vi "Get CustomDevice Reference.vi"(8 "error in":errorcluster, 11 "Node Ptr":T1 format="%.0x") -> (0 "error out":errorcluster, 2 "Custom Device":refnum<k24>, 3 "Node Ptr":T1 format="%.0x")   [LabVIEW 2026, in "Template System Explorer.lvlib"]
uses:
  Template System Explorer.lvlib
  <vilib>/NI VeriStand/Custom Device API/Custom Device Item Ref.ctl
  NationalInstruments.VeriStand.SystemDefinitionAPI
  <vilib>/NI VeriStand/Custom Device API/Custom Device API.lvlib
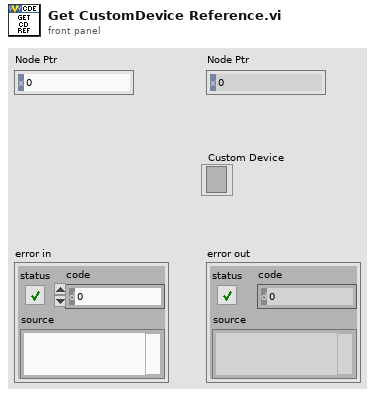
[diagram p1: front panel]
types:
  T1 = typedef "Custom Device API.lvlib/Custom Device Item Ref.ctl" = u64
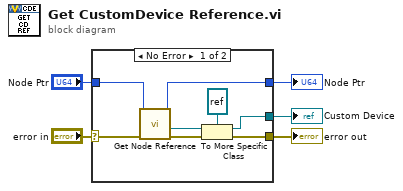
[diagram p0: block diagram]
diagram:
  n1 = case shown="No Error" "error in" {
    selector: "error in" -> [w10 w15]
    tunnel: [w9 w15] -> w4
    tunnel: "Node Ptr" -> [w7 w14]
    tunnel: [w8 w14] -> w2
    tunnel: [w11 _] -> w1
    frame No Error {
      n2 = call "Get Node Reference.vi"("error in"=w10, "Node Ptr"=w7) -> ("error out"=w13:errorcluster, "Base Node"=w6:refnum<k24>, "Node Ptr"=w8:T1)  [unwired: 6 in, 1 out]
      n3 = To More Specific Class(target class=refnum<k24> refnum ("IDToCustomDevice"), reference=w6, error in=w13) -> (specific class reference=w11:refnum<k24>, error out=w9:errorcluster)
    }
    frame Error {
    }
  }
  "error out" <- w4
  "Node Ptr" <- w2
  "Custom Device" <- w1
